vi "Charger_Is One IPG Found.vi"(5 "Status Refnum":T1, 6 "error in":errorcluster, 9 "MICS ID array":u32[](array[numeric]) format="%.0x") -> (0 "error out":errorcluster {"code" format="%.0x"}, 2 "found one IPG":bool, 3 "MICS ID":u32 format="%06x")   [LabVIEW 2020]
doc: "This function displays an \"IPG Shutdown successfully.\" message in the IPG Status cluster."
uses:
  Charger_Status Refnum.ctl
  Drivers/Charger Test Set/Charger_Input Control.ctl
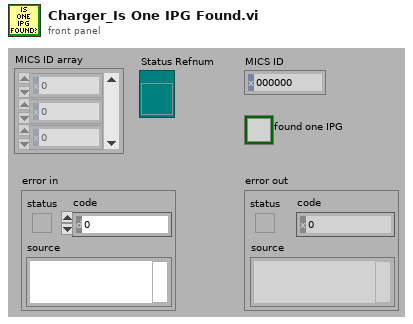
[diagram p1: front panel]
types:
  T1 = typedef "Charger_Status Refnum.ctl" = refnum<vi>
  T2 = typedef "Charger_Input Control.ctl" = cluster{"address":refnum<visa-resource-name>, "position":i32, "setpoint":dbl}
  T3 = cluster{"MICS ID":u32, "VBAT":dbl, "ChargingState":string, "VBAT Slide":dbl, "Status":string, "TemperatureLevel":dbl, "IPG_ReceivedLevel":dbl, "VBAT Target":dbl, "Charger Setpoint":dbl, "Index":i32, "Ready":bool, "Charger Inputs":T2, "MICS Inputs":cluster{"address":refnum<visa-resource-name>, "chan":u16, "ID":u32}}
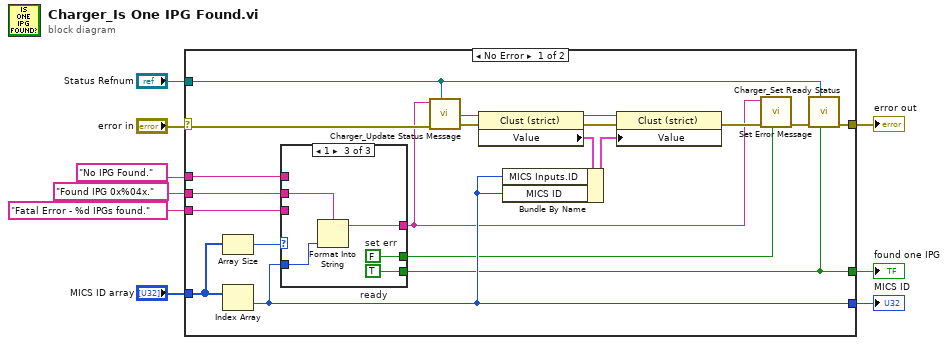
[diagram p0: block diagram]
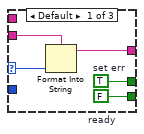
[diagram p2: hidden frame]
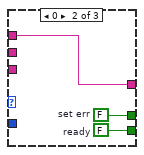
[diagram p3: hidden frame]
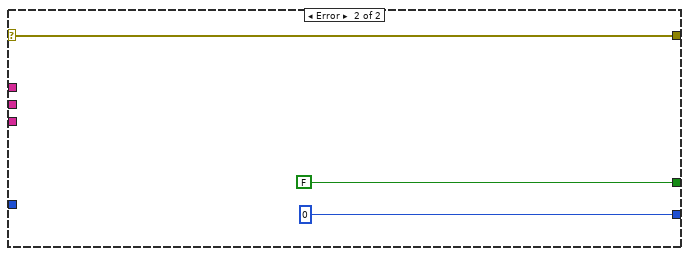
[diagram p4: hidden frame]
diagram:
  n1 = case shown="No Error" "error in" {
    selector: "error in" -> [w27 w44]
    tunnel: [w10 FALSE ("Device Found?")] -> w9
    tunnel: [w13 w44] -> w8
    tunnel: [w21 u32 0 ("Numeric")] -> w7
    tunnel: "Status Refnum" -> [w12 _]
    tunnel: "MICS ID array" -> [w28 _]
    tunnel: "Found IPG 0x%04x." ("Message") -> [w20 _]
    tunnel: "No IPG Found." ("Message") -> [w19 _]
    tunnel: "Fatal Error - %d IPGs found." ("message") -> [w18 _]
    frame No Error {
      n2 = Array Size(array=w28) -> (size(s)=w22:i32)
      n3 = Index Array(array=w28) -> (element=w21:u32)  [unwired: 1 in]
      n4 = case shown="1" w22 {
        selector: w22 -> [w30 _ _]
        tunnel: w21 -> [_ _ w41]
        tunnel: [w33 w35 w40] -> w11
        tunnel: w20 -> [_ _ w37]
        tunnel: [w31 w36 w39] -> w17
        tunnel: w19 -> [_ w36 _]
        tunnel: [w32 w34 w38] -> w10
        tunnel: w18 -> [w29 _ _]
        frame Default {
          w32 = FALSE  # ready
          w33 = TRUE  # set err
          n5 = Format Into String(format string=w29, w30) -> (resulting string=w31:string)  [unwired: 2 in, 1 out]
        }
        frame 0 {
          w34 = FALSE  # ready
          w35 = FALSE  # set err
        }
        frame 1 {
          w38 = TRUE  # ready
          w40 = FALSE  # set err
          n6 = Format Into String(format string=w37, w41) -> (resulting string=w39:string)  [unwired: 2 in, 1 out]
        }
      }
      n7 = call "Charger_Update Status Message.vi"("Status Refnum"=w12, "error in"=w27, "status message"=w17) -> ("error out"=w26:errorcluster)  [unwired: 6 in]
      n8 = property class="Clust (strict)"(reference=w12, error in=w26) -> (reference out=w24:T1, error out=w25:errorcluster, "Value"=w16:T3)
      n9 = Bundle By Name(cluster=w16, "MICS Inputs.ID"=w21, "MICS ID"=w21) -> (w15:T3)
      n10 = property class="Clust (strict)"(reference=w24, error in=w25, "Value"=w15) -> (error out=w23:errorcluster)  [unwired: 1 out]
      n11 = call "Set Error Message.vi"("enable (T)"=w11, "error in"=w23, "message"=w17) -> ("error out"=w14:errorcluster)  [unwired: 5 in]
      n12 = call "Charger_Set Ready Status.vi"("Ready"=w10, "Status Refnum"=w12, "error in"=w14) -> ("error out"=w13:errorcluster)  [unwired: 6 in, 1 out]
    }
    frame Error {
    }
  }
  "error out" <- w8
  "found one IPG" <- w9
  "MICS ID" <- w7
